vi "ex02_front_block.vi"() -> ()   [LabVIEW 2019]
panel:
  in  "Stop Button":bool
  out "Tank":dbl(slide) scale=0.0..100.0
  out "Waveform Chart":dbl(graph)
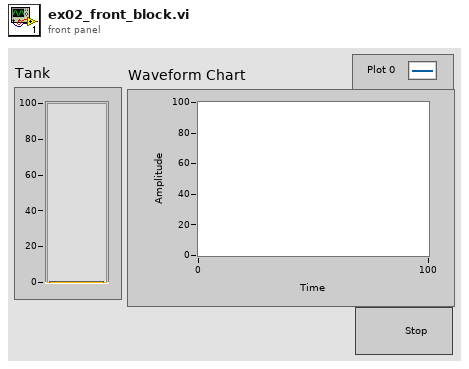
[diagram p1: front panel]
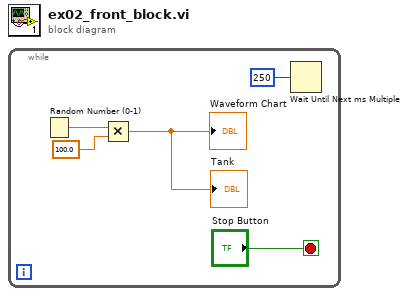
[diagram p0: block diagram]
diagram:
  n1 = while {
    stop <- "Stop Button" stop-if-true
    n2 = Random Number (0-1)() -> (number: 0 to 1=w3:dbl)
    n3 = Multiply(x=w3, y=100.0) -> (x*y=→"Waveform Chart" →"Tank":dbl)
    n4 = Wait Until Next ms Multiple(millisecond multiple=u32 250) -> ()  [unwired: 1 out]
  }
